vi "Vision_Set_Pose.vi"(11 "Vison Pose":T1={"TRANSLATION"={"X"=0.0, "Y"=0.0}, "ROTATION"={"VALUE"=0.0, "COS"=1.0, "SIN"=0.0}} {"ROTATION"."SIN" format="%13.4f"; "ROTATION"."COS" format="%13.4f"; "ROTATION"."VALUE" format="%13.4f"; "TRANSLATION"."Y" format="%14.3f"; "TRANSLATION"."X" format="%14.3f"}) -> ()   [LabVIEW 2023]
uses:
  <vilib>/Rock Robotics/WPI/ThirdParty/JAS_Junk/TrajLib/TypeDef/POSE2D.ctl
  <vilib>/Rock Robotics/WPI/ThirdParty/JAS_Junk/TrajLib/TypeDef/TRANSLATION2D.ctl
  <vilib>/Rock Robotics/WPI/ThirdParty/JAS_Junk/TrajLib/TypeDef/ROTATION2D.ctl
  <vilib>/numeric/Random Number (Range) DBL.vi
  <vilib>/Rock Robotics/WPI/ThirdParty/JAS_Junk/TrajLib/VI/Util_GetTime_U32.vi
  <vilib>/Rock Robotics/WPI/ThirdParty/JAS_Junk/TrajLib/VI/TimeInterpPose2d_CleanUp.vi
  <vilib>/Rock Robotics/WPI/ThirdParty/JAS_Junk/TrajLib/Pose2d_Interpolate.vi
  <vilib>/Rock Robotics/WPI/ThirdParty/JAS_Junk/TrajLib/VI/numCmd_ObtainQueue_Generic.vi
  <vilib>/Rock Robotics/WPI/ThirdParty/JAS_Junk/TrajLib/Twist2d_GetAll.vi
  <vilib>/Rock Robotics/WPI/ThirdParty/JAS_Junk/TrajLib/Twist2d_Create.vi
  <vilib>/Rock Robotics/WPI/ThirdParty/JAS_Junk/TrajLib/VI/Util_GetTime_U64.vi
  <vilib>/gmath/interp.llb/Search Ordered Table.vi
  <vilib>/Rock Robotics/WPI/ThirdParty/JAS_Junk/TrajLib/Pose2d_Log.vi
  <vilib>/Rock Robotics/WPI/ThirdParty/JAS_Junk/TrajLib/Pose2d_Exp.vi
  <vilib>/Rock Robotics/WPI/ThirdParty/JAS_Junk/TrajLib/Trajectory_Library.lvlib
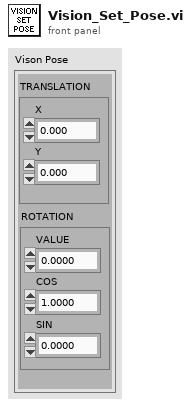
[diagram p1: front panel]
types:
  T1 = typedef "Trajectory_Library.lvlib/POSE2D.ctl" = cluster{"TRANSLATION":T2, "ROTATION":T3}
  T2 = typedef "Trajectory_Library.lvlib/TRANSLATION2D.ctl" = cluster{"X":dbl, "Y":dbl}
  T3 = typedef "Trajectory_Library.lvlib/ROTATION2D.ctl" = cluster{"VALUE":dbl, "COS":dbl, "SIN":dbl}
  T4 = typedef "Trajectory_Library.lvlib/TIME_INTERPOLATABLE_POSE2D.ctl" = cluster{"TimeStamps":dbl[], "Pose":T1[], "Min_TimeStamp":dbl, "Max_TimeStamp":dbl, "ItemCount":i32, "MaxBufferTime":dbl}
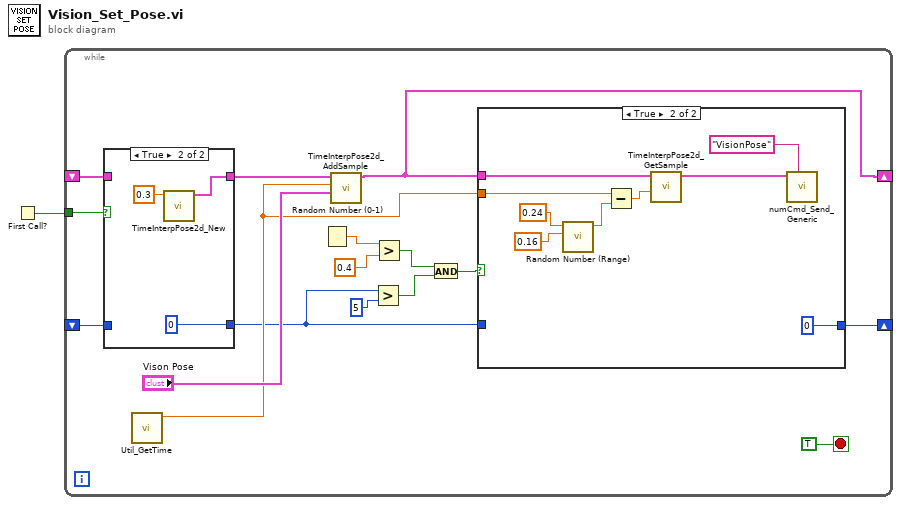
[diagram p0: block diagram]
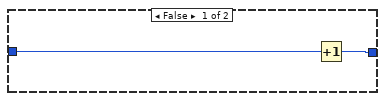
[diagram p2: hidden frame]
diagram:
  n1 = First Call?() -> (First Call?: T/F=w1:bool)
  n2 = while {
    tunnel: w1 -> [w17]
    shift-right: [w9] -> _
    shift-left: _ -> [w15]
    shift-right: [w8] -> _
    shift-left: _ -> [w7]
    stop <- TRUE stop-if-true
    n3 = case shown="True" w17 {
      tunnel: [w30 w32] -> w14
      tunnel: w15 -> [w30 _]
      tunnel: [w29 0] -> w6
      tunnel: w7 -> [w29 _]
      frame False {
      }
      frame True {
        n4 = call <vilib>:"TimeInterpPose2d_New.vi"("MaxTime"=0.3) -> ("TimeInterpPose"=w32:T4)  [unwired: 10 in]
      }
    }
    n5 = call <vilib>:"Util_GetTime.vi"() -> ("FPGA_Time_Seconds"=w10:dbl)  [unwired: 9 in, 2 out]
    n6 = Random Number (0-1)() -> (number: 0 to 1=w12:dbl)
    n7 = call <vilib>:"TimeInterpPose2d_AddSample.vi"("Pose"="Vison Pose", "TimeStamp"=w10, "in TimeInterpPose"=w14) -> ("out TimeInterpPose"=w9:T4)  [unwired: 7 in, 1 out]
    n8 = Greater?(x=w6, y=5) -> (0:w3:bool)
    n9 = Greater?(x=w12, y=0.4) -> (0:w4:bool)
    n10 = And(x=w4, y=w3) -> (x .and. y?=w2:bool)
    n11 = case shown="True" w2 {
      tunnel: w9 -> [_ w28]
      tunnel: w10 -> [_ w25]
      tunnel: [w19 0] -> w8
      tunnel: w6 -> [w18 _]
      frame False {
        n12 = Increment(x=w18) -> (x+1=w19:i32)
      }
      frame True {
        n13 = call-poly <vilib>:"Random Number (Range).vi"("lower bound (0)"=0.16, "upper bound (100)"=0.24) -> ("number"=w24:dbl)  [unwired: 9 in]
        n14 = Subtract(x=w25, y=w24) -> (x-y=w23:dbl)
        n15 = call <vilib>:"TimeInterpPose2d_GetSample.vi"("TimeStamp"=w23, "TimeInterpPose"=w28) -> ("OutputPose"=w21:T1)  [unwired: 8 in, 1 out]
        n16 = call <vilib>:"numCmd_Send_Generic.vi"("Command Name"="VisionPose", "Value"=w21) -> ()  [unwired: 9 in, 1 out]
      }
    }
  }
